vi "enterMaintenance.vi"(8 "error in (no error)":errorcluster, 9 "Parameters":T1, 10 "Model in":refnum<class "Model.lvclass">, 11 "ParkedState in":refnum<class "ParkedState.lvclass">) -> (0 "error out":errorcluster, 2 "Model out":refnum<class "Model.lvclass">, 3 "ParkedState out":refnum<class "ParkedState.lvclass">)   [LabVIEW 2016, in "ParkedState.lvclass"]
uses:
  ParkedState.lvclass
  DataTypes/Topics/CommandEnterMaintenance.ctl
  DataTypes/Topics/Parts/CommandId.ctl
  Model/Model.lvclass
  DataTypes/Topics/Parts/DetailedStates.ctl
  DataTypes/Topics/M1M3SupportTopics.lvlib
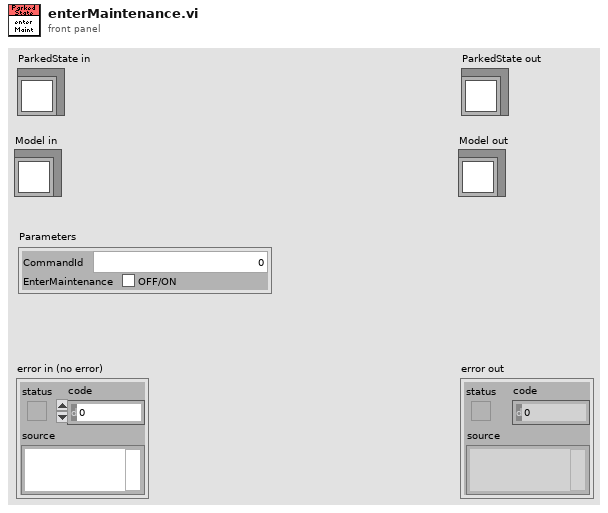
[diagram p1: front panel]
types:
  T1 = typedef "M1M3SupportTopics.lvlib/CommandEnterMaintenance.ctl" = cluster{"CommandId":T2, "EnterMaintenance":bool}
  T2 = typedef "M1M3SupportTopics.lvlib/CommandId.ctl" = i32
  T3 = typedef "M1M3SupportTopics.lvlib/DetailedStates.ctl" = enum16{"OfflineState", "InitialState", "StandbyState", "DisabledState", "ParkedState", "FaultState", "ParkedMaintenanceState", "ActiveMaintenanceState"}
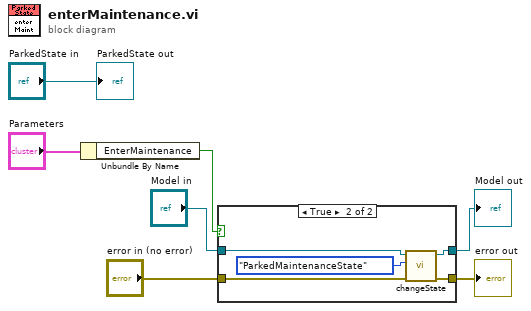
[diagram p0: block diagram]
diagram:
  n1 = Unbundle By Name("Parameters") -> ("EnterMaintenance"=w3:bool)
  n2 = case shown="True" w3 {
    tunnel: "Model in" -> [w9 w14]
    tunnel: [w9 w13] -> w5
    tunnel: [w8 w10] -> w2
    tunnel: "error in (no error)" -> [w8 w11]
    frame False {
    }
    frame True {
      n3 = call "changeState.vi"("error in (no error)"=w11, "DetailedStates"=DetailedStates."ParkedMaintenanceState", "Model in"=w14) -> ("error out"=w10:errorcluster, "Model out"=w13:refnum<class "Model.lvclass">)  [unwired: 7 in]
    }
  }
  "error out" <- w2
  "Model out" <- w5
  "ParkedState out" <- "ParkedState in"
